vi "Addon.Initialize.vi"(8 "error in (no error)":errorcluster, 10 "Diagnostics Basic Configuration":T2, 11 "Device Item Ref in":T1 format="%.0x") -> (0 "error out":errorcluster, 3 "Device Item Ref out":T1=18446744073709551615 format="%.0x")   [LabVIEW 2019, in "Diagnostics Addon System Explorer.lvlib"]
uses:
  Diagnostics Addon System Explorer.lvlib
  Types/Addon.Initialize.ctl
  Addon Shared/Types/Protocol.ctl
  <vilib>/NI VeriStand/Custom Device API/Custom Device Item Ref.ctl
  Addon Shared/SubVIs/Constants.vi
  <vilib>/NI VeriStand/Custom Device Tools/Custom Device Utility Library/NI VeriStand - Search for Item by GUID.vi
  <vilib>/NI VeriStand/Custom Device Tools/Custom Device Utility Library/NI VeriStand - Search for Item by Name.vi
  Addon Shared/Diagnostics Addon Shared.lvlib
  <vilib>/NI VeriStand/Custom Device Tools/Custom Device Utility Library/Custom Device Utility Library.lvlib
  <vilib>/NI/NI VeriStand Custom Device Import and Export Tool/ImportExport.lvlib
  <vilib>/NI VeriStand/Custom Device API/Custom Device API.lvlib
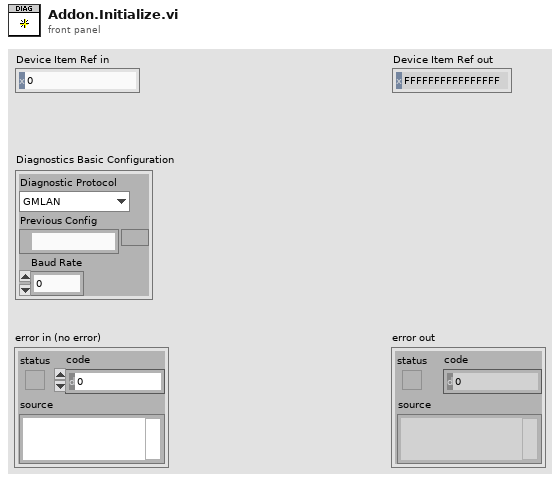
[diagram p1: front panel]
types:
  T1 = typedef "Custom Device API.lvlib/Custom Device Item Ref.ctl" = u64
  T2 = typedef "Diagnostics Addon System Explorer.lvlib/Addon.Initialize.ctl" = cluster{"Diagnostic Protocol":T3, "Previous Config":path, "Baud Rate":u32}
  T3 = typedef "Diagnostics Addon Shared.lvlib/Protocol.ctl" = enum16{"GMLAN", "KWP-2000", "UDS", "User-Defined"}
  T4 = typedef "Diagnostics Addon Shared.lvlib/CAN.ctl" = cluster{"Interface":T5, "Baud Rate":u64, "Diagnostic Protocol":T3, "Transport Protocol":T6, "Transmit ID":u32, "Receive ID":u32, "Transmit Extension":u8, "Receive Extension":u8, "Receive UUDT ID":u32, "Enable Stream":bool, "VW TP Channel ID":u32, "Fill Frame":bool, "Fill Byte":u8, "Termination":bool, "LIN Cluster":refnum<k21>, "NAD":u8, "IO Mode":u32, "Max DLC":u16, "FD Baud Rate":u64, "Timeout":u32, "FD ISO Mode":u32, "DoIP Address":string, "DoIP Source Address":u16, "DoIP Dynamic Port":bool, "DoIP Version":u16}
  T5 = typedef "Diagnostics Addon Shared.lvlib/CAN.Interface.ctl" = string
  T6 = typedef "Diagnostics Addon Shared.lvlib/Transport.ctl" = enum16{"ISO TP - Normal Mode", "ISO TP - Mixed Mode", "VW TP 2.0", "Diagnostics on IP", "ISO TP LIN"}
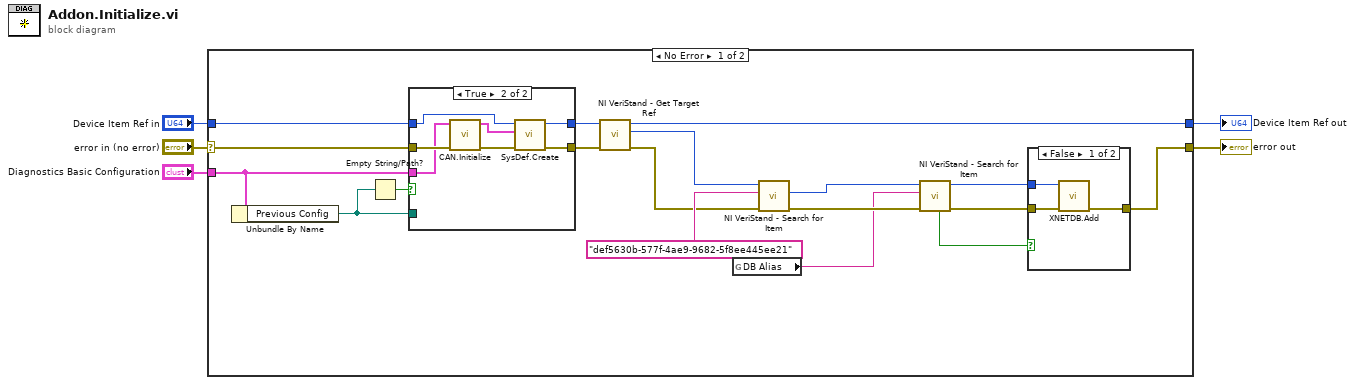
[diagram p0: block diagram]
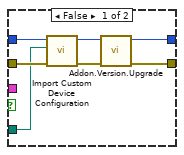
[diagram p2: hidden frame]
diagram:
  n1 = case shown="No Error" "error in (no error)" {
    selector: "error in (no error)" -> [w23 w42]
    tunnel: "Diagnostics Basic Configuration" -> [w21 _]
    tunnel: "Device Item Ref in" -> [w22 w43]
    tunnel: [w8 w43] -> w1
    tunnel: [w18 w42] -> w2
    frame No Error {
      n2 = Unbundle By Name(w21) -> ("Previous Config"=w19:path)
      n3 = Empty String/Path?(string/path=w19) -> (empty?=w20:bool)
      n4 = case shown="True" w20 {
        tunnel: [w24 w31] -> w10
        tunnel: [w26 w32] -> w13
        tunnel: w23 -> [w29 w37]
        tunnel: w22 -> [w30 w33]
        tunnel: w21 -> [_ w36]
        tunnel: w19 -> [w28 _]
        frame False {
          n5 = call <vilib>:"Import Custom Device Configuration.vi"("error in (no error)"=w29, "Path"=w28, "NodeID"=w30) -> ("error out"=w27:errorcluster, "NodeID out"=w25:u64)  [unwired: 6 in, 1 out]
          n6 = call "Addon.Version.Upgrade.vi"("error in (no error)"=w27, "Device Item Ref in in"=w25) -> ("error out"=w26:errorcluster, "Device Item Ref out"=w24:T1)  [unwired: 8 in]
        }
        frame True {
          n7 = call "CAN.Initialize.vi"("error in (no error)"=w37, "Diagnostics Basic Configuration"=w36) -> ("error out"=w35:errorcluster, "Diagnostics Configuration"=w34:T4)  [unwired: 8 in]
          n8 = call "SysDef.Create.vi"("error in (no error)"=w35, "Diagnostics Configuration"=w34, "Device Item Ref in"=w33) -> ("error out"=w32:errorcluster, "Device Item Ref out"=w31:T1)  [unwired: 7 in]
        }
      }
      n9 = call <vilib>:"NI VeriStand - Get Target Ref.vi"("error in"=w13, "Item Ref in"=w10) -> ("error out"=w14:errorcluster, "Target Ref"=w12:T1, "Item Ref out"=w8:T1)  [unwired: 6 in, 1 out]
      n10 = global read "Constants.vi" "DB Alias"() -> (w11:string)
      n11 = call-poly <vilib>:"NI VeriStand - Search for Item.vi"("error in"=w14, "Item GUID"="def5630b-577f-4ae9-9682-5f8ee445ee21" ("string"), "Section Ref in"=w12) -> ("error out"=w15:errorcluster, "Item Ref"=w16:T1)  [unwired: 5 in, 2 out]
      n12 = call-poly <vilib>:"NI VeriStand - Search for Item.vi"("error in"=w15, "Item Name"=w11, "Section Ref in"=w16) -> ("error out"=w9:errorcluster, "Section Ref out"=w7:T1, "Found"=w6:bool)  [unwired: 5 in, 1 out]
      n13 = case shown="False" w6 {
        tunnel: [w40 w41] -> w18
        tunnel: w9 -> [w39 w41]
        tunnel: w7 -> [w38 _]
        frame False {
          n14 = call "XNETDB.Add.vi"("error in (no error)"=w39, "Databases Section Ref"=w38) -> ("error out"=w40:errorcluster)  [unwired: 8 in, 1 out]
        }
        frame True {
        }
      }
    }
    frame Error {
    }
  }
  "error out" <- w2
  "Device Item Ref out" <- w1
